vi "mupDefineConst.vi"(8 "error in (no error)":errorcluster, 9 "Value":dbl, 10 "constName":string, 11 "hParser in":u64) -> (0 "error out":errorcluster, 3 "hParser out":u64)   [LabVIEW 2018, in "mupLib.lvlib"]
doc: "Define a constant and specify its value."
uses:
  mupLib.lvlib
  <vilib>/Utility/error.llb/Error Cluster From Error Code.vi
  libmuparser-lv.dll
panel:
  # "Define a constant and specify its value."
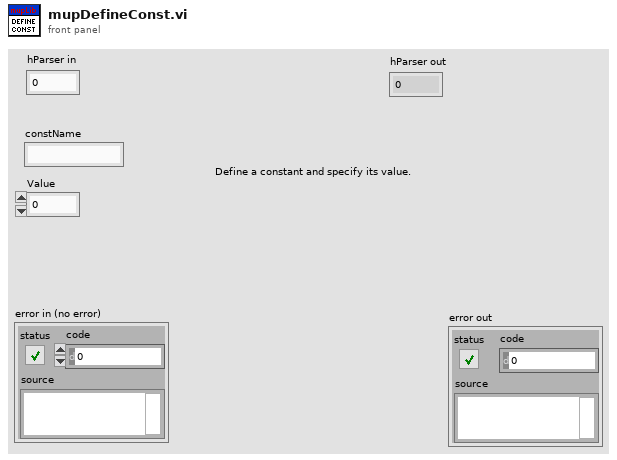
[diagram p1: front panel]
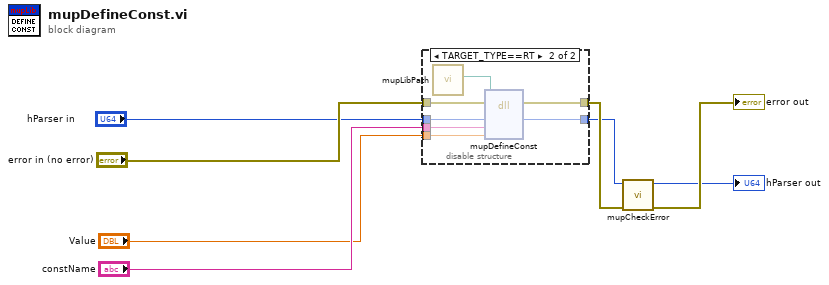
[diagram p0: block diagram]
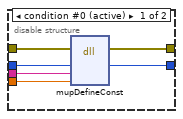
[diagram p2: hidden frame]
diagram:
  n1 = disable-structure shown="TARGET_TYPE==RT" {
    disable-tunnel: "constName" -> [w14 w21]
    disable-tunnel: [w13 w20] -> w7
    disable-tunnel: "error in (no error)" -> [w12 w19]
    disable-tunnel: "Value" -> [w11 w18]
    disable-tunnel: "hParser in" -> [w10 w17]
    disable-tunnel: [w9 w16] -> w1
    frame condition #0 (active) {
      n2 = dll-call lib="C:/Users/leonidas/Documents/GitHub/LV-muParser/mupLib/libmuparser-lv.dll" fn="mupDefineConst"(error in=w12, "hParser"=w10, "szName"=w14, "fVar"=w11) -> (error out=w13:errorcluster, "hParser"=w9:u64)  [unwired: 5 in, 1 out]
    }
    frame condition #1 {
      n3 = call "mupLibPath.vi"() -> ("libmuparser path"=w15:path)  [unwired: 11 in]
      n4 = dll-call lib="C:/Users/leonidas/Documents/GitHub/LV-muParser/mupLib/libmuparser-lv.dll" fn="mupDefineConst"(path in=w15, error in=w19, "hParser"=w17, "szName"=w21, "fVar"=w18) -> (error out=w20:errorcluster, "hParser"=w16:u64)  [unwired: 4 in, 1 out]
    }
  }
  n5 = call "mupCheckError.vi"("error in (no error)"=w7, "hParser in"=w1) -> ("error out"=→"error out":errorcluster, "hParser out"=→"hParser out":u64)  [unwired: 8 in]
